vi "Pcre2Error.vi"(7 "message":string, 9 "error in":errorcluster, 10 "ErrorCode":i32) -> (1 "error out":errorcluster)   [LabVIEW 2021, in "libpcre2-8.lvlib"]
uses:
  libpcre2-8.lvlib
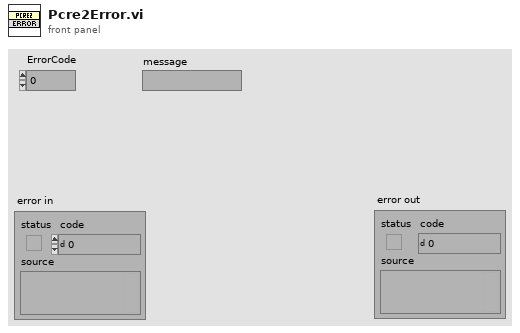
[diagram p1: front panel]
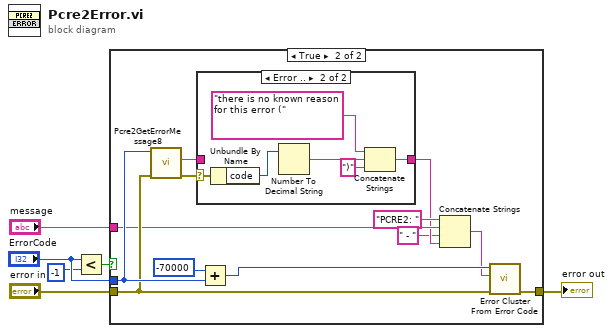
[diagram p0: block diagram]
diagram:
  n1 = Less?(x="ErrorCode", y=-1) -> (x < y?=w4:bool)
  n2 = case shown="True" w4 {
    tunnel: "error in" -> [w7 w15]
    tunnel: [w7 w14] -> w5
    tunnel: "ErrorCode" -> [_ w16]
    tunnel: "message" -> [_ w12]
    frame False {
    }
    frame True {
      n3 = call "Pcre2GetErrorMessage8.vi"("error in"=w15, "ErrorCode"=w16) -> ("error out"=w17:errorcluster, "ErrorMessage"=w18:string)  [unwired: 7 in, 1 out]
      n4 = case shown="Error .." w17 {
        selector: w17 -> [_ w22]
        tunnel: w18 -> [w20 _]
        tunnel: [w20 w26] -> w9
        frame No Error {
        }
        frame Error {
          n5 = Unbundle By Name(w22) -> ("code"=w21:i32)
          n6 = Number To Decimal String(number=w21) -> (decimal integer string=w24:string)  [unwired: 1 in]
          n7 = Concatenate Strings("there is no known reason for this error (" ("ErrorMessage"), w24, ")" ("string")) -> (w26:string)
        }
      }
      n8 = Add(x=-70000 ("errorcode"), y=w16) -> (x+y=w13:i32)
      n9 = Concatenate Strings("PCRE2: " ("string"), w12, " - " ("string"), w9) -> (w11:string)
      n10 = call <vilib>:"Error Cluster From Error Code.vi"("error in (no error)"=w15, "error message (\"\")"=w11, "error code (0)"=w13) -> ("error out"=w14:errorcluster)  [unwired: 6 in]
    }
  }
  "error out" <- w5
